vi "Get Object Parameter - Known Type.vi"(6 "Get Value as JSON Tree? (F)":bool, 8 "error in (no error)":errorcluster, 10 "Parameter Name":string, 11 "JSON Tree In (JSON Object)":variant) -> (0 "error out":errorcluster, 1 "is JSON Null?":bool, 2 "Value":variant, 3 "JSON Tree Passthrough":variant, 5 "JSON Compatible Type":T1=enum."Unknown", 7 "JSON Type":T2=enum."Unknown")   [LabVIEW 2010, in "i3-json.lvlib"]
doc: "Use this template to build a VI to use as a subVI."
uses:
  i3-json.lvlib
  JSON Types/JSON Type.ctl
  JSON Types/JSON Compatible Type.ctl
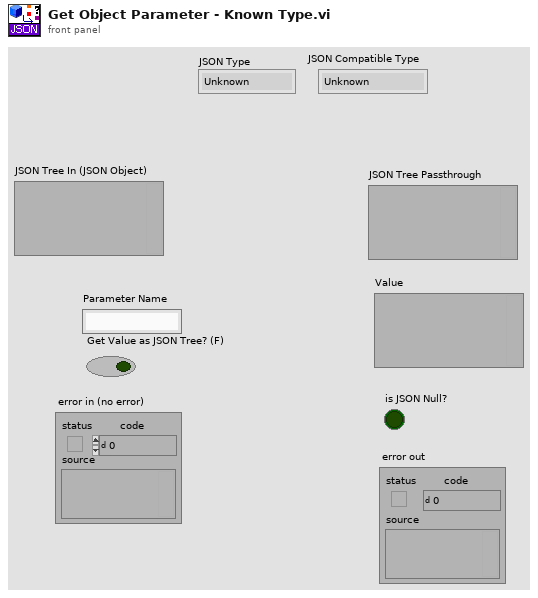
[diagram p1: front panel]
types:
  T1 = typedef "i3-json.lvlib/JSON Compatible Type.ctl" = enum16{"1D Double Array", "1D String Array", "1D Boolean Array", "Unknown"}
  T2 = typedef "i3-json.lvlib/JSON Type.ctl" = enum8{"JSON Compatible", "JSON Array", "JSON Object", "JSON Null", "Double", "String", "Boolean", "Unknown"}
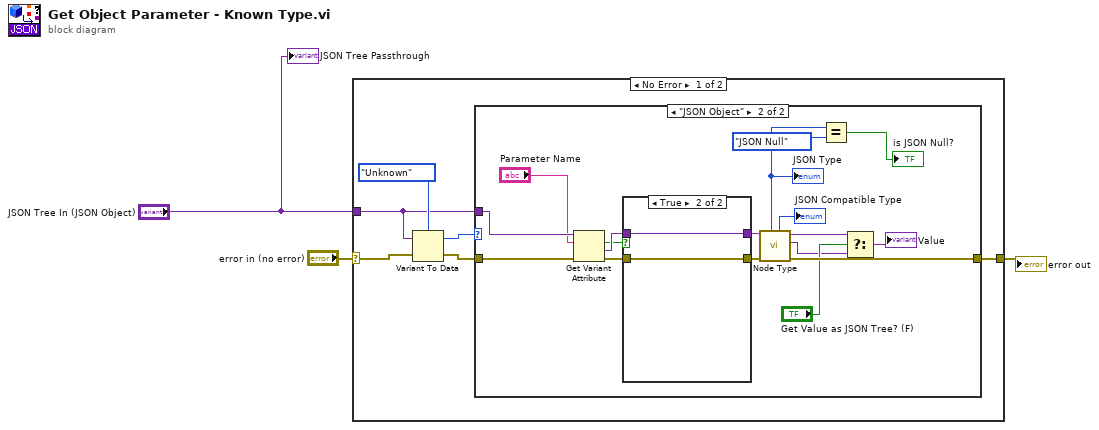
[diagram p0: block diagram]
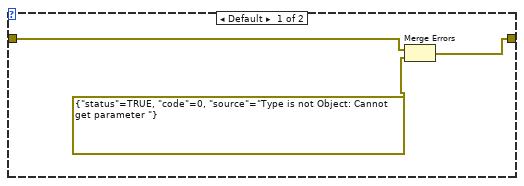
[diagram p2: hidden frame]
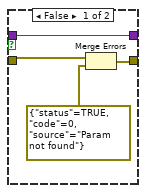
[diagram p3: hidden frame]
diagram:
  n1 = case shown="No Error" "error in (no error)" {
    selector: "error in (no error)" -> [w9 w36]
    tunnel: [w5 w36] -> w2
    tunnel: "JSON Tree In (JSON Object)" -> [w4 _]
    frame No Error {
      n2 = Variant To Data(error in=w9, Variant=w4, type=JSON_Type."Unknown" ("JSON Type")) -> (error out=w7:errorcluster, data=w6:T2)
      n3 = case shown="\"JSON Object\"" w6 {
        tunnel: w7 -> [w11 w29]
        tunnel: w4 -> [_ w28]
        tunnel: [w12 w27] -> w5
        frame Default {
          n4 = Merge Errors(w11, errorcluster {"status"=TRUE, "code"=0, "source"="Type is not Object: Cannot get parameter "} ("error out")) -> (w12:errorcluster)
        }
        frame "JSON Object" {
          n5 = Get Variant Attribute(Variant=w28, name="Parameter Name", error in=w29) -> (found=w20:bool, value=w22:variant, error out=w24:errorcluster)  [unwired: 1 in, 1 out]
          n6 = case shown="True" w20 {
            tunnel: w24 -> [w31 w35]
            tunnel: [w32 w35] -> w23
            tunnel: w22 -> [w33 w34]
            tunnel: [w33 w34] -> w21
            frame False {
              n7 = Merge Errors(w31, errorcluster {"status"=TRUE, "code"=0, "source"="Param not found"} ("error out")) -> (w32:errorcluster)
            }
            frame True {
            }
          }
          n8 = call "Node Type.vi"("error in (no error)"=w23, "JSON Tree In"=w21) -> ("error out"=w27:errorcluster, "Value"=w14:variant, "JSON Tree Passthrough"=w15:variant, "JSON Compatible Type"=→"JSON Compatible Type":T1, "JSON Type"=w19:T2)  [unwired: 5 in]
          "JSON Type" <- w19
          n9 = Equal?(x=w19, y=JSON_Type."JSON Null") -> (x = y?=→"is JSON Null?":bool)
          n10 = Select(t=w15, s="Get Value as JSON Tree? (F)", f=w14) -> (s? t:f=→"Value":variant)
        }
      }
    }
    frame Error {
    }
  }
  "error out" <- w2
  "JSON Tree Passthrough" <- "JSON Tree In (JSON Object)"
